vi "Set - Time Data OBJ.vi"(0 "reference in":refnum<class "AdvSigProc.lvclass">, 5 "error in (no error)":errorcluster, 7 "Time Data":T1) -> (14 "reference out":refnum<class "AdvSigProc.lvclass">, 19 "error out":errorcluster)   [LabVIEW 2020, in "AdvSigProc.lvclass"]
uses:
  AdvSigProc.lvclass
  API/GSwFormDSP_class/GSwFormDSP.lvclass
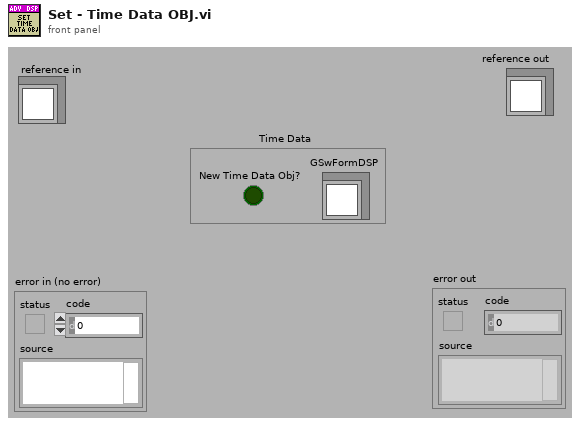
[diagram p1: front panel]
types:
  T1 = cluster{"New Time Data Obj?":bool, "GSwFormDSP":refnum<class "GSwFormDSP.lvclass">}
  T2 = typedef "AdvSigProc.lvclass/ObjectAttributesRef.ctl" = refnum<data-value>
  T3 = typedef "AdvSigProc.lvclass/ObjectAttributes.ctl" = cluster{"Time Data":cluster{"New Time Data Obj?":bool, "GSwFormDSP":refnum<class "GSwFormDSP.lvclass">}, "LMS Parameters":T4}
  T4 = typedef "AdvSigProc.lvclass/LMS.ctl" = cluster{"adaptive filter Ref":refnum<k20>, "Filtered Signals":refnum<class "GSwFormDSP.lvclass">, "Filter Coefs":dbl[], "Input Parameters":T5, "Iteration Metrics":T6[]}
  T5 = typedef "AdvSigProc.lvclass/LMS Input Parameters.ctl" = cluster{"Type":enum16{"Normalized LMS", "LMS", "FIR Sign LMS", "FIR Fast Block LMS", "RLS", "QR - RLS"}, "Filter Class":enum16{"Noise Cancelling (BGN Ref)", "Noise Cancelling (Speech Ref)"}, "Filter Length":i32, "µ Parameters":cluster{"Type":enum16{"User Input", "Auto µ"}, "step size":dbl}, "Iterations":cluster{"Current":i32, "Maximum":i32}}
  T6 = typedef "AdvSigProc.lvclass/Iteration Metrics.ctl" = cluster{"Name":string, "Max":dbl, "Min":dbl, "Values History":dbl[]}
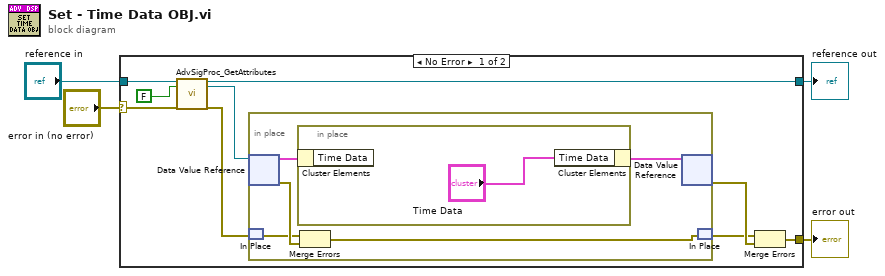
[diagram p0: block diagram]
diagram:
  n1 = case shown="No Error" "error in (no error)" {
    selector: "error in (no error)" -> [w9 w21]
    tunnel: [w13 w21] -> w3
    tunnel: [w8 w20] -> w1
    tunnel: "reference in" -> [w11 w20]
    frame No Error {
      n2 = call "AdvSigProc_GetAttributes.vi"("reference in"=w11, "return data? (T)"=FALSE, "error in (no error)"=w9) -> ("reference out"=w8:refnum<class "AdvSigProc.lvclass">, "attributes ref"=w7:T2, "error out"=w6:errorcluster)  [unwired: 13 in, 1 out]
      n3 = in-place {
        n4 = in-place-dvr #1(w7) -> (w17:T3, w16:errorcluster)
        n5 = in-place-match #2(w6) -> (w15:errorcluster)
        n6 = in-place {
          n7 = in-place-cluster #3(w17) -> ()  [unwired: 1 out]
          n8 = in-place-cluster #3("Time Data"="Time Data") -> (w18:T3)
        }
        n9 = Merge Errors(w15, w16) -> (w14:errorcluster)
        n10 = in-place-dvr #1(w18) -> (w12:errorcluster)  [unwired: 1 out]
        n11 = in-place-match #2(w14) -> (w5:errorcluster)
      }
      n12 = Merge Errors(w5, w12) -> (w13:errorcluster)
    }
    frame Error {
    }
  }
  "error out" <- w3
  "reference out" <- w1
